vi "pulse input.vi"() -> ()   [LabVIEW 2023]
uses:
  <vilib>/DAQmx/read.llb/DAQmx Read (Analog 1D Wfm NChan NSamp).vi
  <vilib>/DAQmx/write.llb/DAQmx Write (Analog 1D Wfm NChan NSamp).vi
  <vilib>/DAQmx/create/channels.llb/DAQmx Create Channel (AI-Voltage-Basic).vi
  <vilib>/DAQmx/configure/timing.llb/DAQmx Timing (Sample Clock).vi
  <vilib>/DAQmx/create/channels.llb/DAQmx Create Channel (AO-Voltage-Basic).vi
  <vilib>/DAQmx/miscellaneous.llb/DAQmx Fill In Error Info.vi
panel:
  out "Waveform Graph 2":waveform(dbl)(graph)
  in  "physical channels 2":tag
  in  "physical channels":tag
  out "Duty Cycle 2":dbl
  out "Period 2":dbl
  out "Frequency 2":dbl
  out "Duty Cycle":dbl
  out "Period":dbl
  out "Frequency":dbl
  out "Waveform Graph":waveform(dbl)(graph)
  in  "stop":bool
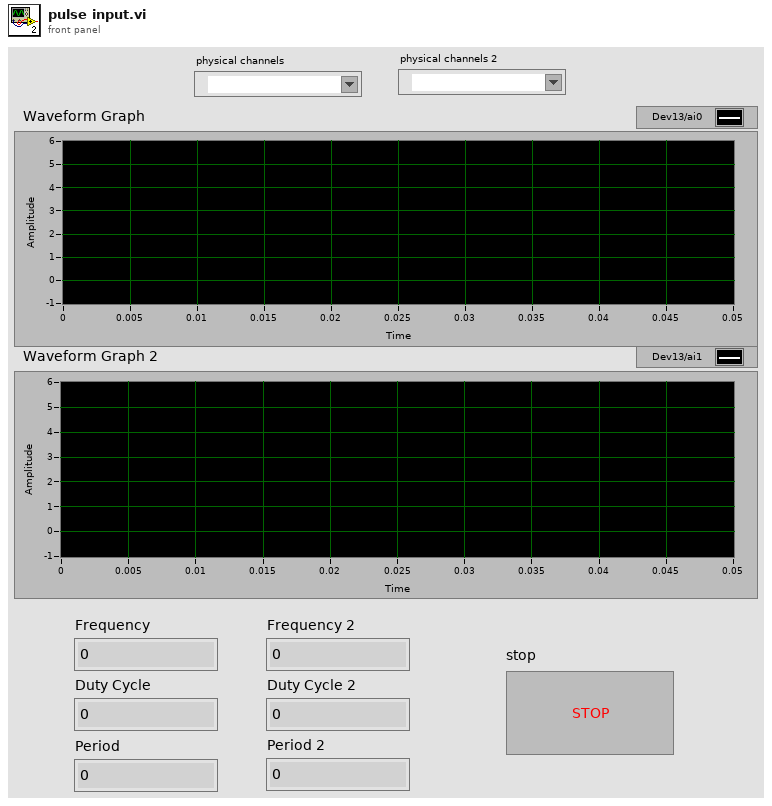
[diagram p1: front panel]
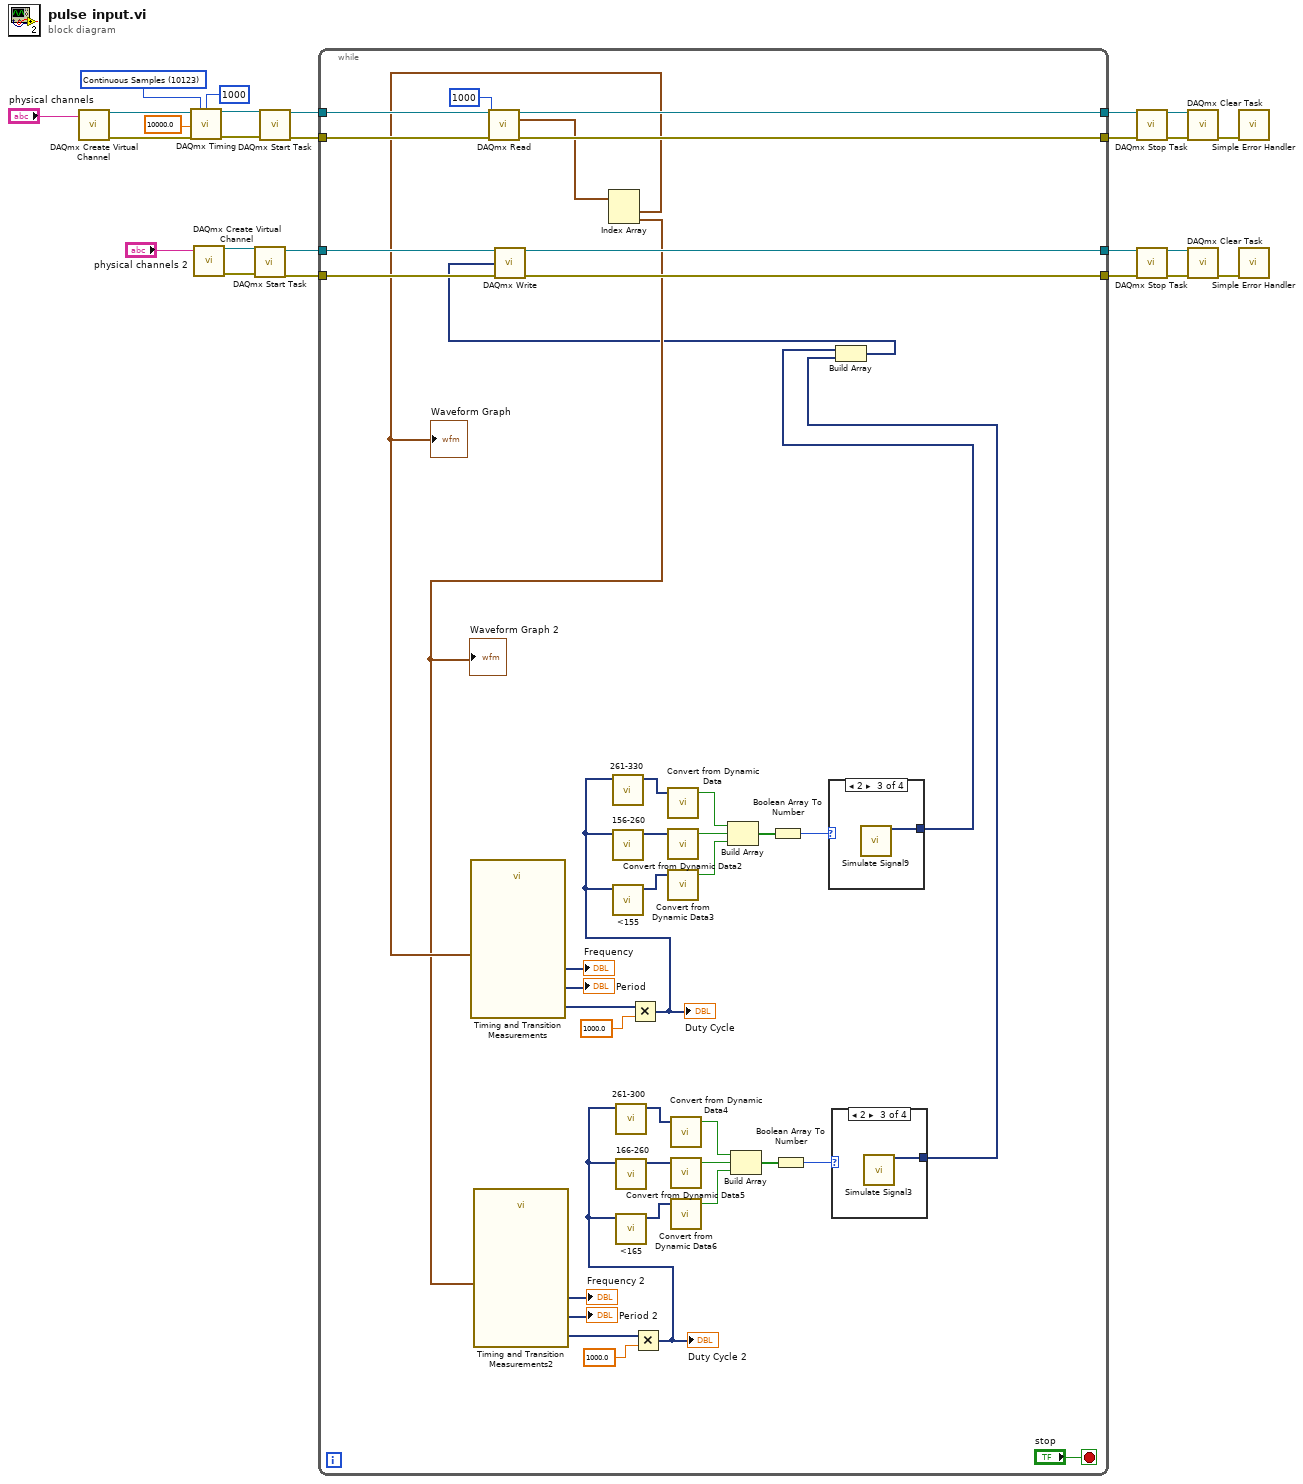
[diagram p0: block diagram]
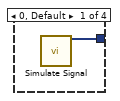
[diagram p2: hidden frame]
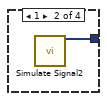
[diagram p3: hidden frame]
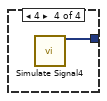
[diagram p4: hidden frame]
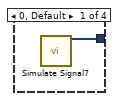
[diagram p5: hidden frame]
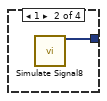
[diagram p6: hidden frame]
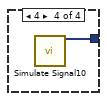
[diagram p7: hidden frame]
diagram:
  w17 = 10123 items=["Finite Samples"=10178, "Continuous Samples"=10123, "Hardware Timed Single Point"=12522] ("sample mode")
  n1 = call-poly <vilib>:"DAQmx Create Virtual Channel.vi"("physical channels"="physical channels") -> ("task out"=w22:refnum<k21>, "error out"=w21:errorcluster)  [unwired: 13 in]
  n2 = call-poly <vilib>:"DAQmx Timing.vi"("task/channels in"=w22, "sample mode"=w17, "samples per channel"=1000, "rate"=10000.0, "error in"=w21) -> ("task out"=w19:refnum<k21>, "error out"=w20:errorcluster)  [unwired: 9 in]
  n3 = call-poly <vilib>:"DAQmx Create Virtual Channel.vi"("physical channels"="physical channels 2") -> ("task out"=w15:refnum<k21>, "error out"=w14:errorcluster)  [unwired: 13 in]
  n4 = call <vilib>:"DAQmx Start Task.vi"("task/channels in"=w15, "error in"=w14) -> ("task out"=w10:refnum<k21>, "error out"=w8:errorcluster)  [unwired: 12 in]
  n5 = call <vilib>:"DAQmx Start Task.vi"("task/channels in"=w19, "error in"=w20) -> ("task out"=w6:refnum<k21>, "error out"=w5:errorcluster)  [unwired: 12 in]
  n6 = while {
    tunnel: w10 -> [w40]
    tunnel: [w39] -> w9
    tunnel: w8 -> [w38]
    tunnel: [w37] -> w7
    tunnel: w6 -> [w35]
    tunnel: [w33] -> w4
    tunnel: w5 -> [w34]
    tunnel: [w32] -> w3
    stop <- "stop" stop-if-true
    n7 = call-poly <vilib>:"DAQmx Read.vi"("task/channels in"=w35, "number of samples per channel"=1000, "error in"=w34) -> ("task out"=w33:refnum<k21>, "data"=w31:waveform(dbl)[], "error out"=w32:errorcluster)  [unwired: 10 in]
    n8 = Index Array(array=w31) -> (element #1=w30:waveform(dbl), element #2=w29:waveform(dbl))  [unwired: 2 in]
    "Waveform Graph" <- w30
    "Waveform Graph 2" <- w29
    n9 = call "Timing and Transition Measurements"("Signals"=w30) -> ("Frequency"=→"Frequency":dynamicdata, "Period"=→"Period":dynamicdata, "Duty Cycle"=w64:dynamicdata)  [unwired: 7 in, 1 out]
    n10 = call "Timing and Transition Measurements2"("Signals"=w29) -> ("Frequency"=→"Frequency 2":dynamicdata, "Period"=→"Period 2":dynamicdata, "Duty Cycle"=w51:dynamicdata)  [unwired: 7 in, 1 out]
    n11 = Multiply(x=w64, y=1000.0) -> (x*y=w62:dynamicdata)
    "Duty Cycle" <- w62
    n12 = call "261-330"("Operand 1"=w62) -> ("Result"=w61:dynamicdata)  [unwired: 9 in, 1 out]
    n13 = call "156-260"("Operand 1"=w62) -> ("Result"=w60:dynamicdata)  [unwired: 9 in, 1 out]
    n14 = call "<155"("Operand 1"=w62) -> ("Result"=w59:dynamicdata)  [unwired: 9 in, 1 out]
    n15 = Multiply(x=w51, y=1000.0) -> (x*y=w49:dynamicdata)
    "Duty Cycle 2" <- w49
    n16 = call "261-300"("Operand 1"=w49) -> ("Result"=w48:dynamicdata)  [unwired: 9 in, 1 out]
    n17 = call "166-260"("Operand 1"=w49) -> ("Result"=w47:dynamicdata)  [unwired: 9 in, 1 out]
    n18 = call "<165"("Operand 1"=w49) -> ("Result"=w46:dynamicdata)  [unwired: 9 in, 1 out]
    n19 = call "Convert from Dynamic Data"("Dynamic Data Type"=w61) -> ("Scalar"=w57:bool)  [unwired: 3 in]
    n20 = call "Convert from Dynamic Data2"("Dynamic Data Type"=w60) -> ("Scalar"=w58:bool)  [unwired: 3 in]
    n21 = call "Convert from Dynamic Data3"("Dynamic Data Type"=w59) -> ("Scalar"=w56:bool)  [unwired: 3 in]
    n22 = call "Convert from Dynamic Data4"("Dynamic Data Type"=w48) -> ("Scalar"=w44:bool)  [unwired: 3 in]
    n23 = call "Convert from Dynamic Data5"("Dynamic Data Type"=w47) -> ("Scalar"=w45:bool)  [unwired: 3 in]
    n24 = call "Convert from Dynamic Data6"("Dynamic Data Type"=w46) -> ("Scalar"=w43:bool)  [unwired: 3 in]
    n25 = Build Array(w57, w58, w56) -> (w55:bool[])
    n26 = Build Array(w44, w45, w43) -> (w42:bool[])
    n27 = Boolean Array To Number(Boolean array=w55) -> (number=w54:u32)
    n28 = Boolean Array To Number(Boolean array=w42) -> (number=w41:u32)
    n29 = case shown="2" w54 {
      tunnel: [w72 w73 w74 w75] -> w28
      frame 0, Default {
        n30 = call "Simulate Signal7"() -> ("DC"=w72:dynamicdata)  [unwired: 14 in, 1 out]
      }
      frame 1 {
        n31 = call "Simulate Signal8"() -> ("Square"=w73:dynamicdata)  [unwired: 14 in, 1 out]
      }
      frame 2 {
        n32 = call "Simulate Signal9"() -> ("Square"=w74:dynamicdata)  [unwired: 14 in, 1 out]
      }
      frame 4 {
        n33 = call "Simulate Signal10"() -> ("DC"=w75:dynamicdata)  [unwired: 14 in, 1 out]
      }
    }
    n34 = case shown="2" w41 {
      tunnel: [w68 w69 w70 w71] -> w27
      frame 0, Default {
        n35 = call "Simulate Signal"() -> ("DC"=w68:dynamicdata)  [unwired: 14 in, 1 out]
      }
      frame 1 {
        n36 = call "Simulate Signal2"() -> ("Square"=w69:dynamicdata)  [unwired: 14 in, 1 out]
      }
      frame 2 {
        n37 = call "Simulate Signal3"() -> ("Square"=w70:dynamicdata)  [unwired: 14 in, 1 out]
      }
      frame 4 {
        n38 = call "Simulate Signal4"() -> ("DC"=w71:dynamicdata)  [unwired: 14 in, 1 out]
      }
    }
    n39 = Build Array(w28, w27) -> (w26:dynamicdata[])
    n40 = call-poly <vilib>:"DAQmx Write.vi"("task/channels in"=w40, "data"=w26, "error in"=w38) -> ("task out"=w39:refnum<k21>, "error out"=w37:errorcluster)  [unwired: 10 in, 1 out]
  }
  n41 = call <vilib>:"DAQmx Stop Task.vi"("task/channels in"=w4, "error in"=w3) -> ("task out"=w25:refnum<k21>, "error out"=w23:errorcluster)  [unwired: 12 in]
  n42 = call <vilib>:"DAQmx Stop Task.vi"("task/channels in"=w9, "error in"=w7) -> ("task out"=w13:refnum<k21>, "error out"=w11:errorcluster)  [unwired: 12 in]
  n43 = call <vilib>:"DAQmx Clear Task.vi"("task in"=w25, "error in"=w23) -> ("error out"=w24:errorcluster)  [unwired: 13 in]
  n44 = call <vilib>:"DAQmx Clear Task.vi"("task in"=w13, "error in"=w11) -> ("error out"=w12:errorcluster)  [unwired: 13 in]
  n45 = call <vilib>:"Simple Error Handler.vi"("error in (no error)"=w24) -> ()  [unwired: 4 in, 5 out]
  n46 = call <vilib>:"Simple Error Handler.vi"("error in (no error)"=w12) -> ()  [unwired: 4 in, 5 out]
